vi "Solve2.vi"(8 "Error In":errorcluster, 11 "object in":refnum<class "2022_1.lvclass">) -> (0 "Error Out":errorcluster, 2 "Result":u64, 3 "object out":refnum<class "2022_1.lvclass">)   [LabVIEW 2020, in "2022_1.lvclass"]
uses:
  2022_1.lvclass
  2022_1.lvclass/2022_1.ctl
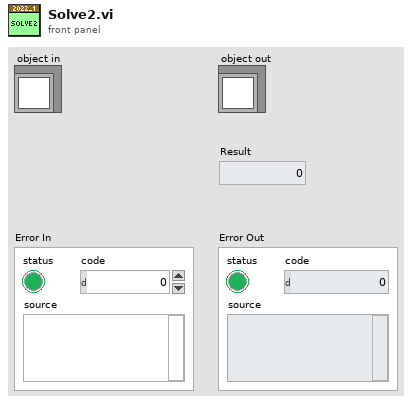
[diagram p1: front panel]
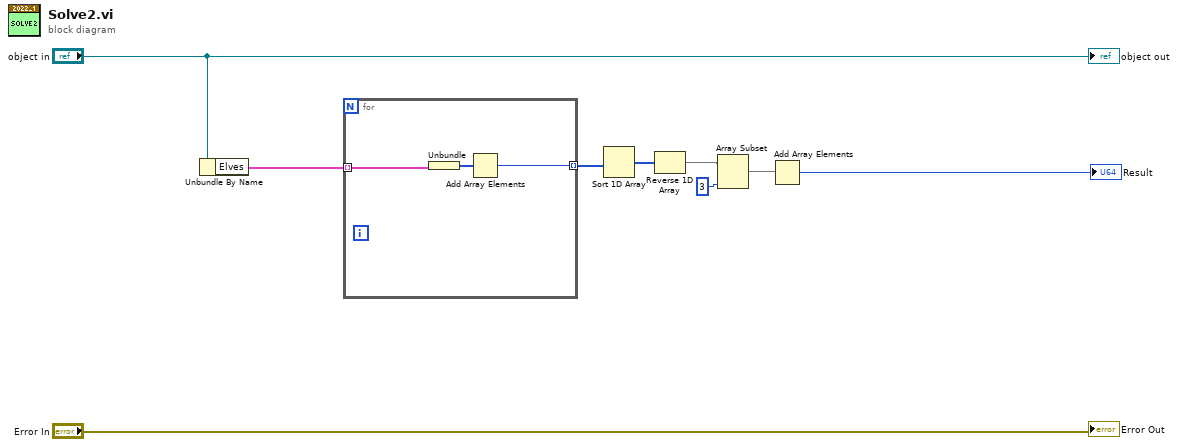
[diagram p0: block diagram]
diagram:
  n1 = Unbundle By Name("object in") -> ("Elves"=w6:cluster{"Calories":u64[]}[])
  n2 = for {
    tunnel: w6 -> [w12] mode=indexing
    tunnel: [w10] -> w5 mode=indexing
    n3 = Unbundle(w12) -> ("Calories"=w11:u64[])
    n4 = Add Array Elements(numeric array=w11) -> (sum=w10:u64)
  }
  n5 = Sort 1D Array(array=w5) -> (sorted array=w4:u64[])
  n6 = Reverse 1D Array(array=w4) -> (reversed array=w3:u64[])
  n7 = Array Subset(array=w3, length=3) -> (w1:u64[])  [unwired: 1 in]
  n8 = Add Array Elements(numeric array=w1) -> (sum=→"Result":u64)
  "Error Out" <- "Error In"
  "object out" <- "object in"
